vi "Update Graphs.vi"(8 "error in (no error)":errorcluster, 9 "Cursor.Cursor Position":T1, 10 "image":variant[][](array[variant]), 11 "Detail Graph in":refnum<class "Detail Graph.lvclass">) -> (0 "error out":errorcluster, 3 "Detail Graph out":refnum<class "Detail Graph.lvclass">)   [LabVIEW 2023, in "Detail Graph.lvclass"]
uses:
  Detail Graph.lvclass
  Detail Graph.lvclass/Detail Graph.ctl
  Base Graph/Base Graph.lvclass
  D:/git/Graph-Classes/Base Graph/Base Graph.lvclass
  D:/git/Graph-Classes/Detail Graph/Detail Graph.lvclass
  <vilib>/Utility/miscctls.llb/LVPointDoubleTypeDef.ctl
panel:
  in  "Image #":u16
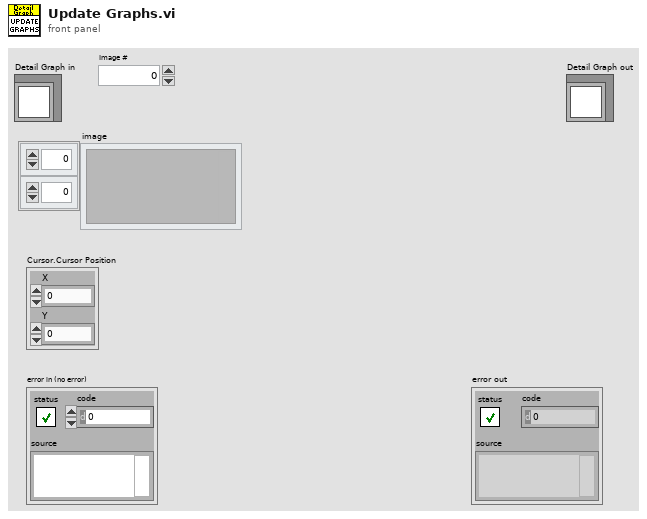
[diagram p1: front panel]
types:
  T1 = typedef "LVPointDoubleTypeDef.ctl" = cluster{"X":dbl, "Y":dbl}
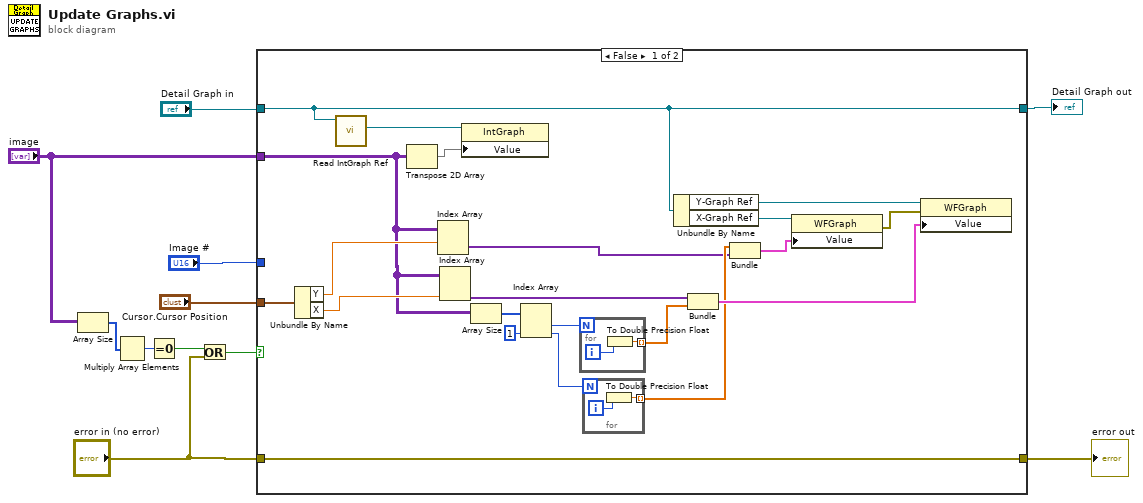
[diagram p0: block diagram]
diagram:
  n1 = Array Size(array="image") -> (size(s)=w4:i32[])
  n2 = Multiply Array Elements(1:w4) -> (0:w7:i32)
  n3 = Equal To 0?(x=w7) -> (x = 0?=w5:bool)
  n4 = Or(x=w5, y="error in (no error)") -> (x .or. y?=w6:bool)
  n5 = case shown="False" w6 {
    tunnel: [w14 w37] -> w11
    tunnel: [w20 w38] -> w1
    tunnel: "Detail Graph in" -> [w20 w38]
    tunnel: "Cursor.Cursor Position" -> [w32 _]
    tunnel: "Image #" -> [_ _]
    tunnel: "image" -> [w21 _]
    tunnel: "error in (no error)" -> [w14 w37]
    frame False {
      n6 = Unbundle By Name(w32) -> ("Y"=w27:dbl, "X"=w24:dbl)
      n7 = call "Read IntGraph Ref.vi"("TG Base Graph in"=w20) -> ("IntGraph Ref"=w31:refnum<vi>)  [unwired: 8 in, 2 out]
      n8 = Transpose 2D Array(2D array=w21) -> (transposed array=w28:variant[][])
      n9 = Index Array(array=w21, index (row)=w27) -> (element=w12:variant[])  [unwired: 1 in]
      n10 = Index Array(array=w21, index (col)=w24) -> (element=w22:variant[])  [unwired: 1 in]
      n11 = property class="IntGraph"(reference=w31, "Value"=w28) -> ()  [unwired: 1 in, 2 out]
      n12 = Array Size(array=w21) -> (size(s)=w30:i32[])
      n13 = Index Array(array=w30, index #2=1 ("index")) -> (element #1=w29:i32, element #2=w25:i32)  [unwired: 1 in]
      n14 = for {
        N: w29 -> [_]
        tunnel: [w36] -> w23 mode=indexing
        i -> [w35]
        n15 = To Double Precision Float(number=w35) -> (double precision float=w36:dbl)
      }
      n16 = for {
        N: w25 -> [_]
        tunnel: [w33] -> w13 mode=indexing
        i -> [w34]
        n17 = To Double Precision Float(number=w34) -> (double precision float=w33:dbl)
      }
      n18 = Unbundle By Name(w20) -> ("Y-Graph Ref"=w19:refnum<vi>, "X-Graph Ref"=w17:refnum<vi>)
      n19 = Bundle("image"=w22, w23) -> (w15:cluster{"image":variant[], dbl[]})  [unwired: 1 in]
      n20 = Bundle(w13, "image"=w12) -> (w16:cluster{dbl[], "image":variant[]})  [unwired: 1 in]
      n21 = property class="WFGraph"(reference=w17, "Value"=w16) -> (error out=w18:errorcluster)  [unwired: 1 in, 1 out]
      n22 = property class="WFGraph"(reference=w19, error in=w18, "Value"=w15) -> ()  [unwired: 2 out]
    }
    frame True {
    }
  }
  "error out" <- w11
  "Detail Graph out" <- w1
